vi "Build.vi"(8 "error in (no error)":errorcluster, 11 "Task in":refnum<class "Task.lvclass">) -> (0 "error out":errorcluster, 1 "Build Specification Version":T1, 2 "Generated files":path[](array[path]), 3 "Task out":refnum<class "Task.lvclass">)   [LabVIEW 2017, in "Task Interface.lvlib" / "Task.lvclass"]
uses:
  Task.lvclass
  <vilib>/AppBuilder/AB_API_Simple/Build Specification Version.ctl
  Task.lvclass/Task.ctl
  <vilib>/AppBuilder/AB_API_Simple/Build (path).vi
  <vilib>/AppBuilder/AB_API_Simple/NI_App_Builder_API.lvlib
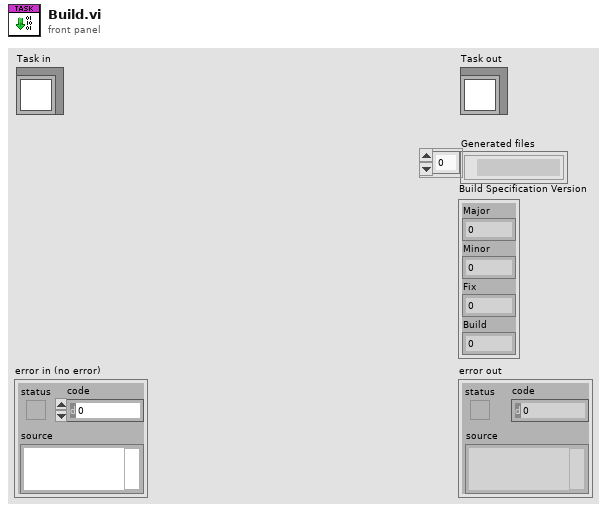
[diagram p1: front panel]
types:
  T1 = typedef "NI_App_Builder_API.lvlib/Build Specification Version.ctl" = cluster{"Major":u16, "Minor":u16, "Fix":u16, "Build":u16}
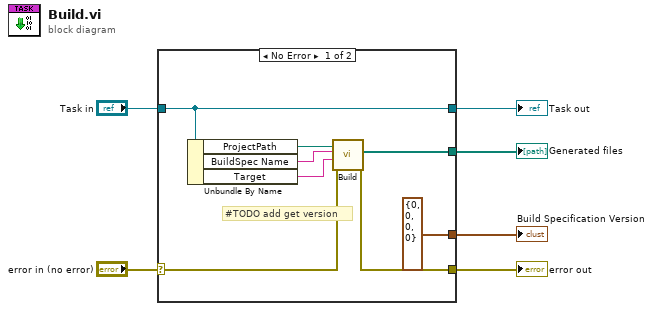
[diagram p0: block diagram]
diagram:
  n1 = case shown="No Error" "error in (no error)" {
    selector: "error in (no error)" -> [w13 w16]
    tunnel: [w8 w16] -> w5
    tunnel: [w14 w15] -> w3
    tunnel: "Task in" -> [w14 w15]
    tunnel: [w12 _] -> w2
    tunnel: [T1 {"Major"=0, "Minor"=0, "Fix"=0, "Build"=0} ("Build Specification Version") _] -> w1
    frame No Error {
      # "#TODO add get version"
      n2 = Unbundle By Name(w14) -> ("ProjectPath"=w11:path, "BuildSpec Name"=w10:string, "Target"=w9:string)
      n3 = call-poly <vilib>:"Build.vi"("error in (no error)"=w13, "Name of target (My Computer)"=w9, "Name of build specification (if empty: build all)"=w10, "Path to project"=w11) -> ("error out"=w8:errorcluster, "Generated files"=w12:path[])  [unwired: 6 in]
    }
    frame Error {
    }
  }
  "error out" <- w5
  "Task out" <- w3
  "Generated files" <- w2
  "Build Specification Version" <- w1
